vi "Actor Core.vi"(8 "error in":errorcluster, 11 "Test Executive Builder Active Info View In":refnum<class "Test Executive Builder Active Info View.lvclass">) -> (0 "error out":errorcluster, 3 "Actor out":refnum<class "Actor.lvclass">)   [LabVIEW 2017, in "Test Executive Builder Active Info View.lvclass"]
doc: "(<B>Filename</B>: Actor Framework.lvlib:Actor.lvclass:Actor Core.vi)\n\nReceives messages to the actor, reacts to them, and initiates any error handling that may shut the actor down.\n\nDescendant classes may override this VI to append parallel tasks for the actor to complete while it handles messages. Overrides use the Call Parent Method node.\n\n<License>\nCopyright © 2017 Composed Systems, LLC | All rights reserved\nwww.composed.io\n\nAuthor: Ethan Stern <ethan.stern@composed.io>\n\nThis software is provided \"AS IS\" WITHOUT WARRANTIES, either express or implied, AND IS FOR EDUCATIONAL PURPOSES ONLY.\n</License>"
uses:
  Test Executive Builder Active Info View.lvclass
  <vilib>/gpm_packages/@cs/mva-viewable/Source/IViewManager/IViewManager/IViewManager.lvclass
  <vilib>/gpm_packages/@cs/mva-viewable/Source/IViewable/ProtectedSubpanel/ProtectedSubpanel.lvclass
  <vilib>/ActorFramework/Actor/Actor.lvclass
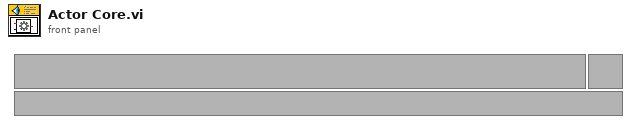
[diagram p1: front panel]
types:
  T1 = typedef "IViewable.lvlib/ProtectedSubpanel.lvclass/Protected Subpanel Reference.ctl" = refnum<data-value>
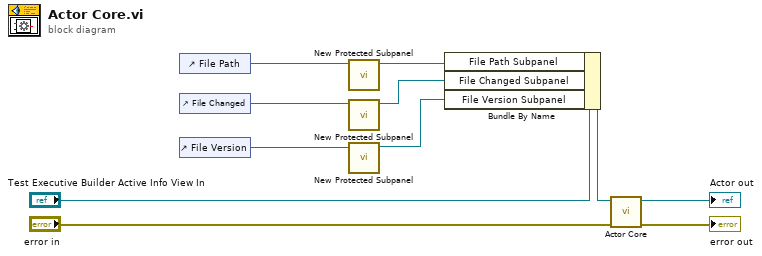
[diagram p0: block diagram]
diagram:
  n1 = control-ref of="File Path"() -> (w5:refnum<vi>)
  n2 = control-ref of="File Changed"() -> (w4:refnum<vi>)
  n3 = control-ref of="File Version"() -> (w2:refnum<vi>)
  n4 = call <vilib>:"New Protected Subpanel.vi"("SubPnl Refnum"=w5) -> ("Protected Subpanel"=w6:T1)  [unwired: 9 in, 1 out]
  n5 = call <vilib>:"New Protected Subpanel.vi"("SubPnl Refnum"=w4) -> ("Protected Subpanel"=w3:T1)  [unwired: 9 in, 1 out]
  n6 = call <vilib>:"New Protected Subpanel.vi"("SubPnl Refnum"=w2) -> ("Protected Subpanel"=w1:T1)  [unwired: 9 in, 1 out]
  n7 = Bundle By Name(cluster="Test Executive Builder Active Info View In", "File Path Subpanel"=w6, "File Changed Subpanel"=w3, "File Version Subpanel"=w1) -> (w7:refnum<class "Test Executive Builder Active Info View.lvclass">)
  n8 = call-parent "Actor Core.vi"("error in"="error in", "IViewable In"=w7) -> ("error out"=→"error out":errorcluster, "Actor out"=→"Actor out":refnum<class "Actor.lvclass">)  [unwired: 8 in]
